vi "UNITEST MAIN v2.0.vi"() -> ()   [LabVIEW 2025]
uses:
  Traction Loop/Traction Receipe Enum.ctl
  controls/LAB-IQ UI Data.ctl
  <vilib>/Platform/TimedLoop/XDataNode/timing_clust.ctl
  <vilib>/Platform/TimedLoop/XDataNode/nitl_modes.ctl
  <vilib>/Platform/TimedLoop/XDataNode/wakeup.ctl
  HEAVE vi's/Heave Write enum.ctl
  SWAY vi's/Sway Write enum.ctl
  Traction Loop/Traction Write enum.ctl
  Acquostics Loops/Write Main Enum.ctl
  SWAY vi's/Sway Right enum.ctl
  HEAVE vi's/Heave Right enum.ctl
  Traction Loop/Traction Read enum.ctl
  Acquostics Loops/Read Main Enum.ctl
  0f9b3d6c-7caf-4790-9f98-5fac89a3677b.vi
  48f5795f-33f4-4366-aaa7-704d1097ecc1.vi
  d081153b-36ca-4bc4-8478-749476f82ba4.vi
  1202965f-721d-4349-8d61-5de826f379ef.vi
  785ec975-e53d-4ed4-be48-2cc128d7a91f.vi
  02c5850b-52e8-4ed5-91f8-6f0ad62f4994.vi
  1223eb78-e4c4-4b69-bf80-185c82055158.vi
  e5651a45-6a49-4a3f-b503-ff1eaf449b4a.vi
  <vilib>/Utility/error.llb/Trim Whitespace One-Sided.vi
  support/Message Queue/Enqueue Message (Single).vi
  <vilib>/Utility/error.llb/Error Cluster From Error Code.vi
  <vilib>/Utility/file.llb/Read Delimited Spreadsheet (string).vi
  <vilib>/Utility/file.llb/Write Delimited Spreadsheet (string).vi
  <vilib>/ErrorRing/Error Ring.xnode
  <vilib>/platform/TimedLoop/XDataNode/XDataNode.xnode
  support/Message Queue/LAB-IQ Message Queue.lvlib
  support/User Event - Stop/LAB-IQ User Event - Stop.lvlib
  <vilib>/Platform/TimedLoop/XDataNode/XDNodeRunTimeDep.lvlib
panel:
  in  "Uplink Traction":refnum<vi>
  in  "Traction":bool
  in  "Scratch":bool
  in  "LRM CAM":bool
  in  "Sway LRM":bool
  in  "Rotary Horizontal":bool
  in  "Rotary Vertical":bool
  in  "Load Cell 2":refnum<vi>
  out "AE Ring-Down Counts":u32(graph)
  out "Signal Energy":sgl(graph)
  out "Amplitude db_AE":sgl(graph)
  out "Peak Amplitude":sgl(graph)
  out "SET entrainment Velocity":dbl
  out "Test Array Size":i32
  in  "SRR INDEX [ STRIBECK]":i32
  out "Stribeck Size":i32
  out "SET SRR":dbl
  out "Enum - READ":T1
  out "ELAPSED TIMER":dbl
  out "BALL SET RPM":dbl
  out "DISC SET RPM":dbl
  out "SET LOAD":dbl
  in  "TEMPERATURE READ":dbl=40.0
  out "SET TEMPERATURE":dbl
  out "Traction Size":i32
  out "DISC SPEED (rpm)":dbl=100.0 min=0.1 max=3000.0 step=0.1 format="%.1f"
  out "BALL SPEED (rpm)":dbl=100.0 min=0.1 max=3000.0 step=0.1 format="%.1f"
  in  "BALL WEAR TRACK":dbl=7.9
  in  "DISC WEARTRACK":dbl=24.0
  in  "SRR INDEX [ TRACTION]":i32
  in  "Start Index Type":i32
  in  "Enum - Menu":T1
  out "Ball (mm/sec)":dbl
  out "Disc (mm/sec)":dbl
  in  "Traction Receipe Update Details":bool
  in  "HomeTraction":bool
  in  "Demo Mode Display":enum32{"Page 1", "Page 2"}(tab)
  in  "Traction Message":string="Recommended motion directions \nfor traction module.\n\nBall:  Counterclockwise\nDisc: Clockwise"
  in  "Traction Step Update Details":bool
  in  "Main Tab sequence for selection":T2(tab)
  out "ExceedDiscSpeed  Cinstant Speed":string
  out "ExceedBallSpeed Constant":string
  in  "TEST SELECTION (MTM) 2":enum32{"Ball Speed", "Disc Speed"}(radio)
  in  "SPEED SELECTION : MTM 2":enum32{"Speed in Rpm", "Speed in m/sec"}(radio)=enum."Speed in m/sec"
  in  "MTM Test Selection 2":enum32{"Time", "Cycle"}(radio)
  in  "Enter the Speed (m/sec):":dbl=0.5 min=3e-06 max=2500.0 step=0.001 format="%.6f"
  in  "Enter the Speed (m/sec):":dbl=0.5 min=3e-06 max=3000.0 step=0.001 format="%.6f"
  in  "Enter the Speed (RPM):":dbl=100.0 min=0.1 max=3000.0 step=0.1 format="%.1f"
  out "Lower Spped":string
  out "Upper":string
  in  "Enter the Speed (RPM):":dbl=1.0 min=0.1 max=2500.0 step=0.1 format="%.1f"
  out "ExceedBallSpeed step":string
  out "ExceedDiscSpeed":string
  out "Disc Speed Indicator":bool
  out "ExceedBallSpeed":string
  out "BallSpeed Exceed Indication":bool
  in  "Apply":bool
  in  "SPEED SELECTION : MTM":enum32{"Speed in Rpm", "Speed in m/sec"}(radio)=enum."Speed in m/sec"
  in  "TEST SELECTION (MTM)":enum32{"Ball Speed", "Disc Speed"}(radio)
  in  "MTM Test Selection":enum32{"Time", "Cycle"}(radio)
  in  "File Path Tab":enum32{"Page 1", "Page 2"}(tab)
  in  "File Path String":string="File Path Location : C:-->LAB-IQ 150 --> User Defined\n                                       Protocol-->File.txt"
  in  "Save":bool
  in  "Import":bool
  in  "File Path :":path
  in  "Step Sequence Indication Tab":enum32{"Page 1", "Page 2"}(tab)
  in  "Step Sequence Indication":string="Minimum 2 Steps required to perform the Speed Sequence"
  in  "Calculate Step":bool
  in  "StepTable":string[][](table)
  in  "Ramp Tab":enum32{"Page 1"}(tab)
  out "e.v/ssr":enum32{"E.V", "SSR"}(tab)
  in  "Enter Fixed SRR":dbl=1.0 min=-1.0 max=1.0 step=0.001 format="%.3f"
  in  "Enter the Final E.Velocity (m/s)":dbl=1.0 min=0.001 max=10.0 step=0.001 format="%.3f"
  in  "Enter initial E.Velocity (m/s)":dbl=2.0 min=0.001 max=10.0 step=0.001 format="%.3f"
  in  "Enter Fixed E.Velocity":dbl=1.0 min=0.001 max=2.0 step=0.001 format="%.3f"
  in  "Enter Final SRR":dbl=1.0 min=-1.0 max=1.0 step=0.001 format="%.2f"
  in  "Enter initial SRR":dbl=1.0 min=-1.0 max=1.0 step=0.001 format="%.2f"
  in  "Ball WTD":dbl=17.32 min=17.32 max=17.32 step=0.001 format="%.2f"
  in  "E.Velocity":bool caption="SRR"
  in  "Enter the Final Velocity (m/s)":dbl=1.0 min=0.001 max=2.0 step=0.001 format="%.3f"
  in  "Enter initial Velocity (m/s)":dbl=2.0 min=0.001 max=2.0 step=0.001 format="%.3f"
  out "Ramp Up   Disc":bool caption="Ramp Down"
  out "Initial DiscSpeed (RPM)":dbl=100.0 min=0.1 max=3000.0 step=0.1 format="%.1f"
  out "Final Speed (RPM)":dbl=1.0 min=0.1 max=3000.0 step=0.1 format="%.1f"
  out "Final Speed (RPM)":dbl=1.0 min=0.1 max=3000.0 step=0.1 format="%.1f"
  out "Initial Speed (RPM)":dbl=100.0 min=0.1 max=3000.0 step=0.1 format="%.1f"
  in  "Enter the Final Velocity (m/s)":dbl=1.0 min=0.001 max=2.0 step=0.001 format="%.3f"
  in  "Enter initial Velocity (m/s)":dbl=2.0 min=0.001 max=2.0 step=0.001 format="%.3f"
  out "Ramp Up":bool caption="Ramp Down"
  in  "Disc Motion Direction:":u16(ring) items=["Clockwise", "Counter Clockwise"]
  in  "Ball Motion Direction :":u16(ring) items=["Clockwise", "Counter Clockwise"]
  in  "Motion Mode:":u16(ring) items=["Uniform Rotation", "Speed Step", "Speed Ramp", "Speed Recipe"]
  in  "Wear Track Diameter (mm) 3":dbl=16.0 caption="Wear Track Diameter (mm):" min=1.0 max=20.0 step=0.01 format="%.2f"
  in  "Set WTD 2":bool
  in  "SRR Sweep Range (%)":string caption="Speed (mm/s)"
  out "Traction Receipe":i32(listbox)=-1
  in  "Total Execution Time":dbl
  in  "Total Steps":dbl
  in  "Duration / Step (s)":dbl=6.0
  in  "STRIBECK Fixed SRR List (%)":string="5,10,20,40,60,80,100"
  in  "Duration / Step (s)":dbl=6.0
  in  "SRR Sweep Range (%)":string
  in  "Speed (mm/s)":dbl=1000.0
  in  "Temperature Stages (°C)":string="40,100,140"
  in  "Load (N)":string="25"
  in  "Lubricant Name":string
  in  "Profile File Name":string
  out "error out":errorcluster
  in  "DEPTH TRIP   ENABLE":bool
  in  "DEPTH TRIP VALUE":dbl
  in  "LOAD TRIP  ENABLE":bool
  in  "LOAD TRIP VALUE":dbl
  in  "CYCLIC COF TRIP  ENABLE":bool
  in  "CYCLIC FF TRIP  ENABLE":bool
  in  "FF TRIP  ENABLE":bool
  in  "COF TRIP  ENABLE":bool
  in  "CYCLIC CoF TRIP VALUE":dbl
  in  "CYCLIC FF TRIP VALUE":dbl
  in  "FF TRIP VALUE":dbl
  in  "COF TRIP VALUE":dbl
  in  "Gain 2":dbl=0.016
  in  "Offset  3":dbl=1.5
  in  "Ramp MulFac":dbl=2.0
  out "actpid":dbl
  in  "pulses LoadDiffRamp(2..10)":dbl=9.0
  in  "PulseControlRamp(diff<=3N)":dbl=5.0 min=1.0 max=1000.0 step=1.0 format="%#.1f"
  in  "SetLoadDeadband(%) Load(0-10N)":dbl=0.1 min=0.0001 max=100.0 step=0.0001 format="%#.6f"
  in  "pulses LoadDiff(2..10)":dbl=10.0
  in  "pulses LoadDiff(11..50)":dbl=40.0
  in  "PulseControl(diff<=3N)":dbl=1.0 min=1.0 max=1000.0 step=1.0 format="%#.1f"
  out "SetLoadDeadband(%)  2":dbl=1.0 min=0.001 max=100.0 step=0.001 format="%#.6f"
  in  "pulsesSent":dbl=200.0
  out "pulses":dbl
  in  "pulses LoadDiff(21..1000)":dbl=40.0
  in  "Delay":dbl=1.5 min=0.001 max=5.0 step=0.001 format="%#.6f"
  in  "deadband":dbl=0.2
  in  "Checkbox 2":bool
  in  "Checkbox":bool=TRUE
  out "Scratch Start Recording":bool
  in  "SwaySpeed Set":bool
  in  "Update":bool
  in  "Analysis Home":bool
  in  "Installation/Replacement completed":bool
  in  "Loahead":bool
  in  "Heave and Surge COM Port:":refnum<visa-resource-name>="COM9"
  in  "Sway COM Port:":refnum<visa-resource-name>="COM10"
  out "Test Trip":bool
  out "Hymidity":bool
  in  "Humidity Disable trip":bool=TRUE
  in  "CoF Trip  2":dbl=540.0 min=100.0 max=540.0 step=1.0
  in  "File Path :  2":path
  out "Wear Track Diameter":dbl
  in  "Stribeck table":bool
  in  "seq":bool=TRUE
  out "Drive Error":string
  out "mm/s  Surge":dbl=7.0 caption="Jog" min=0.001 max=50.0 step=0.0001 format="%.2f"
  in  "Update Surge Speed":bool
  out "mm/s  Sway":dbl=7.0 caption="Jog" min=0.001 max=50.0 step=0.0001 format="%.2f"
  in  "Update Sway Speed":bool
  in  "Update Heave Speed":bool
  out "mm/s Heave":dbl=7.0 caption="Jog" min=0.001 max=30.0 step=0.0001 format="%.2f"
  in  "mm/sec":dbl=1.0 caption="Jog" min=0.001 max=50.0 step=0.001 format="%.2f"
  out "Scratch Start Test":bool
  in  "HomeScratch":bool
  in  "TEST SELECTION":enum32{"Time", "Cycle"}(radio)
  out "Spare 15":u8
  out "Spare 14":u8
  out "Spare 13":u8
  out "Spare 12":u8
  out "Spare 11":u8
  out "Spare 10":u8
  out "Spare 9":u8
  out "Spare 8":u8
  out "Start Test Temp":bool
  in  "AppLoadSeq scratch":bool
  in  "PID Delay (sec)":dbl=1.0 format="%#_6p"
  out "Spare 15":u8
  out "Spare 14":u8
  out "Spare 13":u8
  out "Spare 12":u8
  out "Spare 11":u8
  out "Spare 10":u8
  out "Spare 9":u8
  out "Spare 8":u8
  out "Load Cell Temp":bool
  in  "Stop Scratch":bool
  in  "Enter Fixed SRR 2":dbl min=0.0 max=0.0 format="%.3f"
  in  "E.Velocity 2":bool=TRUE caption="SRR"
  in  "Tab Control 3":T3(tab)
  in  "Tab Control 14":T4(tab)=enum."Motor Load"
  in  "Ramp":bool
  in  "PID":T5={"min_deadband_floor"=50000000.0, "min_finetune_floor"=10.0, "dynamic_spindle_noise_scalar"=100.0, "filter_alpha"=0.05, "Vertical load (N)"=0.0, "Pulse delta"=0.0, "Fine Tune Zone"=10.0, "Max_pos_limit"=50000000.0, "Min_pos_limit"=0.0, "i_limit"=10.0, "Max Step Linit"=10.0, "Init Step"=10.0, "pct_scale"=100.0, "Deadband"=0.1, "Kd"=0.0, "Ki"=0.0, "Kp"=1.0, "Current Position"=0.0, "Set Load"=0.0, "Current Load"=0.0, "gFF Rot 7"={0.0, 0.0, 0.0}, "Bypass Load"=FALSE, "Enter ByPass Load"=0.0, "apply load"=FALSE} {"Vertical load (N)" format="%#.3f"}
  in  "deleteHandle-result":i32
  in  "initial-return":i32
  in  "filter-return":i32
  in  "zero-return":i32
  in  "get-range-return":i32
  in  "get-data-return":i32
  in  "ft_udp_handle":i32
  in  "AE":bool
  in  "reinit 3":bool=TRUE
  in  "AutoTune":bool
  in  "Dummy Run":bool
  in  "running_flag":bool
  in  "Create Handle":bool=TRUE
  in  "delete Handle":bool
  in  "ft_range":dbl[](array[numeric])=[1.0, 1.0, 1.0, 1.0, 1.0, 1.0]
  in  "ft_data":dbl[](array[numeric])=[1.0, 1.0, 1.0, 1.0, 1.0, 1.0]
  in  "PID gains out delay (microForce)":T6={"proportional gain (Kc)"=300.0, "integral time (Ti, min)"=0.00011, "derivative time (Td, min)"=0.0} {"derivative time (Td, min)" format="%.3f"; "integral time (Ti, min)" min=1e-05 max=100.0 step=1e-06 format="%.6f"; "proportional gain (Kc)" format="%.3f"}
  in  "PID gains out delay":T6={"proportional gain (Kc)"=30.0, "integral time (Ti, min)"=0.00101, "derivative time (Td, min)"=0.0} {"derivative time (Td, min)" format="%.3f"; "integral time (Ti, min)" min=1e-05 max=100.0 step=0.0001 format="%.4f"; "proportional gain (Kc)" format="%.3f"}
  in  "output range delay":cluster{"output high":dbl, "output low":dbl}={"output high"=100.0, "output low"=-100.0} {"output low" format="%.2f"; "output high" format="%.2f"}
  in  "Load(N)":dbl[](array[numeric])
  in  "FFy(N)":dbl[](array[numeric])
  in  "FFx(N)":dbl[](array[numeric])
  in  "Mx(Nm)":dbl[](array[numeric])
  in  "My(Nm)":dbl[](array[numeric])
  in  "Mz(Nm)":dbl[](array[numeric])
  in  "Port":i32=8080
  in  "Sensor IP":string="192.168.1.100"
  in  "SN":i32
  in  "model":string
  in  "Burst Delay (ms)":dbl=10.0
  in  "Acq Delay (ms)":dbl=10.0
  in  "ZeroAll":bool
  in  "ClearAll":bool
  in  "Save Dwell":dbl=0.015 caption="Save Dwell (sec)" min=0.0 max=5.0 step=0.001 format="%.3f"
  out "TORQUE (N-m)":dbl[][](graph)
  out "FORCE (N)":dbl[][](graph)
  in  "stop 6":bool
  in  "Tab Control 19":enum32{"Platform COM", "Config ", "DevInfo"}(tab)=enum."Config "
  in  "Manual Write Acquostic":bool
  out "data out":string
  out "Last Config Rejected":u32
  out "rx command count":u32
  out "Current Filter Id":u32
  out "Isolated Gain":u32
  out "DAQ Status":u32
  out "Heave and Surge Read":string
  out "error out Write":errorcluster
  out "error out Read":errorcluster
  out "Read Heave Temp":bool
  out "Heave and Surge Write":string
  in  "Manual Write Heave & Surge":bool
  out "HEAVE ENABLE":bool
  out "SWAY READ":string
  out "error out Write  SWAY":errorcluster
  out "error out Read SWAY":errorcluster
  out "Read SWAY Temp":bool
  out "SWAY WRITE":string
  in  "Manual Write SWAY":bool
  out "TRACTION READ":string
  out "error out Write  TRACTION":errorcluster
  out "error out Read TRACTION":errorcluster
  out "Read TRACTION Temp":bool
  out "TRACTION WRITE":string
  in  "Manual Write TRACTION":bool
  in  "Uplink Packet":T7
  out "Downlink Packet":T8
  in  "error in (no error)":errorcluster
  out "error out":errorcluster
  in  "UPLINK HEAVE":T9={"Sequence ID"=0, "Mode Command"=2, "Distance"=10000.0, "SPEED"=10000.0, "Reserved"=0.0, "SPARE 1"=0, "SPARE 2"=0, "SPARE 3"=0, "SPARE 4"=0, "SPARE 5"=0, "SPARE 6"=0, "SPARE 7"=0, "SPARE 8"=0, "SPARE 9"=0, "SPARE 10"=0, "SPARE 11"=0, "SPARE 12"=0, "SPARE 13"=0, "SPARE 14"=0, "SPARE 15"=0, "SPARE 16"=0, "SPARE 17"=0}
  out "DOWNLINK HEAVE":T10 {"HEAVE POSE" format="%#.6f"; "SURGE POSE" format="%#.6f"; "Missed Packets" format="%#.6f"}
  in  "UPLINK SWAY":T11={"Sequence ID"=0, "Mode Command"=2, "Distance"=10000.0, "SPEED"=10000.0, "Reserved"=0.0, "SPARE1"=0, "SPARE 2"=0, "SPARE  3"=0, "SPARE  4"=0, "SPARE  5"=0, "SPARE 6"=0, "SPARE 7"=0, "SPARE 8"=0, "SPARE 9"=0, "SPARE 10"=0, "SPARE 11"=0, "SPARE 12"=0, "SPARE 13"=0, "SPARE 14"=0, "SPARE 15"=0, "SPARE 16"=0, "SPARE 17"=0}
  out "DOWNLINK SWAY":T12 {"SWAY POSE" format="%#.6f"; "Rotary POSE" format="%#.6f"; "Missed Packets" format="%#.6f"}
  in  "Uplink Traction":T13={"Sequence ID"=0, "Mode Command"=2, "Distance"=10000.0, "SPEED"=10000.0, "Reserved "=0.0, "SPARE 1"=0, "SPARE 2"=0, "SPARE  3"=0, "SPARE  4"=0, "SPARE  5"=0, "SPARE 6"=0, "SPARE 7"=0, "SPARE 8"=0, "SPARE 9"=0, "SPARE 10"=0, "SPARE 11"=0, "SPARE 12"=0, "SPARE 13"=0, "SPARE 14"=0, "SPARE 15"=0, "SPARE 16"=0, "SPARE 17"=0}
  out "Downlink traction":T14 {"TRACTION POSE 1" format="%#.6f"; "TRACTION POSE 2" format="%#.6f"; "Missed Packets" format="%#.6f"}
  in  "JOG TRIP LOAD VALUE (N)":dbl
  in  "SAMPLES":dbl=100.0
  in  "Re-initilaize":bool
  in  "Filter ON/OFF":bool=TRUE
  in  "TracHomeSurgeOffsetCounts 10MM":dbl=505100.0
  in  "TracHomeSwayOffsetCounts 10MM":dbl=1432.0
  in  "Acoustic Emission:":dbl=1.0 min=0.0001 max=200.0 step=0.0001 format="%.4f"
  in  "Apply Filter (FF)":bool
  in  "Filter% 2":dbl=50.0 min=50.0 max=100.0 step=0.1 format="%.1f"
  in  "Apply Filter (Load)":bool=TRUE
  in  "Filter%":dbl=80.0 min=50.0 max=100.0 step=0.1 format="%.1f"
  in  "Sway distance (mm)":dbl=245.0
  in  "Surge distance (mm)":dbl=370.0
  in  "DataSavingLoopDelay(ms)":dbl=15.0
  in  "SAVE  2":bool
  in  "Enter Distance":bool caption="Enter Counts"
  in  "Sway Counts:":dbl=100.0 min=0.0 max=100000000.0 step=1.0 format="%.2f"
  in  "Distance (mm): 3":dbl=100.0 caption="Distance (mm):" min=0.0 max=1500.0 step=0.001 format="%.5f"
  in  "Surge Counts:":dbl=100.0 min=0.0 max=100000000.0 step=1.0 format="%.1f"
  in  "Distance (mm): 2":dbl=100.0 caption="Distance (mm):" min=0.0 max=1500.0 step=0.0001 format="%.3f"
  in  "Distance (mm):":dbl=100.0 min=0.0 max=1500.0 step=0.001 format="%.5f"
  in  "Heave Counts:":dbl=100.0 min=0.0 max=100000000.0 step=1.0
  in  "LRMHomeSurgeOffsetCounts":dbl=307197.0
  in  "LRMHomeSwayOffsetCounts":dbl=26880.0
  in  "TracHomeSurgeOffsetCounts 20MM":dbl=505100.0
  in  "TracHomeSwayOffsetCounts 20MM":dbl=1432.0
  in  "RotHomeSwayOffsetCounts":dbl=14656.0
  in  "RotHomeSurgeOffsetCounts":dbl=311465.0
  in  "Heave distance":dbl=340.0
  out "Zmm":dbl=1600.0
  out "Heave Pulses/mm":dbl=1600.0
  out "Surge Pulses/mm":dbl=1600.0
  out "Sway Pulses/mm":dbl=320.0
  in  "Heave Pitch":dbl=4.0
  in  "Surge Pitch":dbl=3.0
  in  "Sway Pitch":dbl=2.0
  in  "Heave PPR":dbl=6400.0
  in  "Surge PPR":dbl=6400.0
  in  "Sway PPR":dbl=6400.0
  in  "Heave Jog Speed":dbl=15.0
  in  "Surge Jog Speed":dbl=1.0 format="%.4f"
  in  "Heave PID Speed":dbl=15.0
  in  "Heave Loop Delay":dbl
  in  "Sway Jog Speed":dbl=1.0 format="%.4f"
  in  "Sway PID Speed":dbl=1.0 format="%.4f"
  in  "Sway Loop Delay":dbl
  in  "GUI":T15(tab)
  in  "Platform Settings":bool caption="Password"
  in  "Configure":bool caption="Password"
  in  "Home":bool caption="Password"
  in  "EXIT":bool
  in  "Analysis":bool caption="Password"
  in  "service 2":bool caption="Password"
  in  "MainPage":T16(tab)=enum."HOME"
  in  "Select Load Head":bool
  in  "Notes :":string
  in  "FILE":string
  in  "Sample ID :":string
  in  "Operator ID :":string
  in  "Operator Name :":string
  in  "Auto":bool caption="Power Status"
  in  "Disable Axis Jog Soft Limits m":bool
  out "Sway and Surge COM Status":bool=TRUE caption="Load COM Status"
  out "Heave COM Status":bool=TRUE caption="Load COM Status"
  in  "Enable Platform":bool
  in  "Surge Forward Main":bool
  in  "Surge Backward Main":bool
  in  "Sway Right Main":bool
  in  "Sway Left Main":bool
  in  "Heave Down Main":bool
  in  "Heave Up main":bool
  in  "mm":dbl=0.001 caption="Jog" min=0.001 max=30.0 step=0.01 format="%#.3f"
  in  "Surface Analysis":bool
  in  "Imaging":bool
  in  "Image Analysis":bool
  in  "Post Analysis":bool
  in  "SSP 0.75":bool
  in  "SSP 0.5":bool
  in  "SSP 0.3":bool
  in  "Warning":enum32{"Page 2"}(tab)
  in  "gui GIF":enum32{"Check", "Deca", "kilo", "Micro"}(tab)
  out "Communication is established":bool=TRUE caption="Load COM Status"
  in  "Reference Sample":u16(ring) items=["None", "Brass", "Aluminium", "Mild Steel"]
  out "Load Cell Communication Slide":u8(slide)=1 min=1 max=10 step=1 scale=0.0..10.0
  in  "com 3":bool
  out "com":bool
  out "DecaForce COM Status":bool caption="Load COM Status"
  in  "Loading Mode":u16(ring) items=["Constant", "Ramp", "Steps", "Indentation"]
  in  "Enter the CoF Trip":dbl=1.0
  in  "Enter the Friction Force Trip":dbl=520.0 min=500.0 max=500.0 step=1.0 format="%#.1f"
  in  "Enter the Normal load Trip":dbl=520.0 min=500.0 max=500.0 step=0.001 format="%.3f"
  in  "KiloForce":bool
  in  "DecaForce":bool
  in  "MicroForce":bool
  in  "LHBack":bool
  in  "LHNext":bool
  in  "Load Selection":T17(tab)
  in  "Enter the Load  (N)":dbl=2.0 caption="Enter the Load (N)" min=2.0 max=50.0 step=0.1 format="%#.4f"
  in  "Enter the Final Load (N)":dbl=1.0 min=0.0 max=500.0 step=1.0 format="%#.0f"
  in  "Enter the Loading Rate (N/min)":dbl=60.0 min=1.0 max=1200.0 step=0.1 format="%.2f"
  out "Warning 2":bool
  in  "Stribeck Table  For loading":string[][](table)
  in  "Clear 3":bool
  out "Message":string="Load Entered is out of range!!!"
  in  "Indentation":string[][](table)=[["Detection", "5", "2"], ["Unload", "0", "5"], ["Load", "10", "2"], ["Unload", "0", "5"], ["Detection", "5", "2"], ["Unload", "0", "5"]]
  in  "Multipoint":bool caption="Singlepoint"
  in  "AppLoad 4":bool
  in  "zNL":bool
  out "NL disp":dbl caption="Normal Load ( N )" min=-2000.0 max=2000.0 step=0.0001 format="%.1f"
  in  "Traction":bool
  in  "Surge Forward MM":bool
  in  "Surge Backward MM":bool
  in  "M3 Image":enum32{"Page 1", "Page 2"}(tab)
  in  "String 39":string="Jog heave to bring the upper sample closer to the lower sample within 1mm."
  in  "Sway Left MM":bool
  in  "Sway Right MM":bool
  in  "Disable Axis Jog Soft Limits":bool
  in  "mm":dbl=0.001 caption="Jog" min=0.001 max=5.0 step=0.0001 format="%#.3f"
  in  "Heave Down MM":bool
  in  "Heave Up MM":bool
  in  "Wear Track Diameter (mm)":dbl=30.0 caption="Wear Track Diameter (mm):" min=1.0 max=30.0 step=1.0 format="%.2f"
  in  "Set WTD":bool
  in  "HomeScratch":bool
  in  "HomeRot":bool
  in  "PlaceModule":bool
  in  "Motion Mode:":u16(ring) items=["Uniform Rotation", "Angular Oscillation", "Stribeck ", "Steps"]
  in  "LR Sway":bool
  in  "Rot Hor":bool
  in  "Rot Ver":bool
  in  "Scratch":bool
  in  "LR Cam":bool
  in  "MMBack":bool
  in  "MMNext":bool
  in  "Rotary Module Selection":T18(tab)
  in  "SPEED SELECTION :":enum32{"Speed in RPM", "Speed in m/sec"}(radio)=enum."Speed in m/sec"
  in  "Enter the Speed(mm/sec)":dbl=0.1 min=0.0001 max=1000.0 step=0.1 format="%#.4f"
  in  "Enter the Speed (RPM)":dbl=45.0 min=1.0 max=3000.0 step=1.0
  in  "Enter the Frequency (Hz)":dbl=1.0 min=0.1 max=10.0 step=0.1 format="%.1f"
  in  "Enter the Angle (Deg)":dbl=45.0 min=5.0 max=300.0 step=1.0
  in  "Angular Oscillation Set":bool
  in  "Rotary Tab":enum32{"Page 1", "Page 2"}(tab)
  out "e.v/ssr 2":enum32{"E.V", "SSR"}(tab)
  in  "Enter the Final E.Velocity (m/s) 2":dbl=1.0 min=0.001 max=4.0 step=0.001 format="%.3f"
  in  "Enter initial E.Velocity (m/s) 2":dbl=2.0 min=0.001 max=4.0 step=0.001 format="%.3f"
  in  "Enter Fixed E.Velocity 2":dbl=1.0 min=0.001 max=2.0 step=0.001 format="%.3f"
  in  "Enter Final SRR 2":dbl=1.0 min=0.001 max=1.0 step=0.001 format="%.2f"
  in  "Enter initial SRR 2":dbl=1.0 min=0.001 max=1.0 step=0.001 format="%.2f"
  out "Final Speed (RPM) 3":dbl=1.0 min=0.1 max=3000.0 step=0.1 format="%.1f"
  out "Initial Speed (RPM) 2":dbl=100.0 min=0.1 max=3000.0 step=0.1 format="%.1f"
  in  "Enter the Final Velocity (m/s) 3":dbl=1.0 min=0.001 max=2.0 step=0.001 format="%.3f"
  in  "Enter initial Velocity (m/s)  3":dbl=2.0 min=0.001 max=2.0 step=0.001 format="%.3f"
  out "Ramp Up 2":bool caption="Ramp Down"
  in  "Import 2":bool
  in  "Save 2":bool
  in  "SPEED SELECTION : rotary":enum32{"Speed in Rpm", "Speed in m/sec"}(radio)=enum."Speed in m/sec"
  in  "calculate rotary":bool
  in  "String 45":string="File Path Location : C:-->LAB-IQ 150 --> User Defined\n                                       Protocol-->File.txt"
  in  "Step Speed":enum32{"Step Speed", "Step (load-Speed)"}(tab)
  in  "StepTable For Speed":string[][](table)
  in  "StepTable For Load-Speed":string[][](table)=[["", "", ""], ["", "", ""], ["", "", ""], ["", "", ""]]
  in  "StepTable For Speed 3":string[][](table)=[["", "", ""], ["", "", ""], ["", "", ""], ["", "", ""]]
  in  "Motion Direction:  3":u16(ring) items=["Clockwise", "Counter Clockwise"]
  in  "Enter Scratch length (mm):":dbl=1.0 min=1.0 max=50.0 step=0.0001 format="%.4f"
  in  "Enter Scratch Speed (mm/s):":dbl=1.0 min=0.003 max=10.0 step=0.0031 format="%.5f"
  in  "Scartch Offset":dbl=1.0 caption="Scratch Offset: (mm)" min=0.1 max=5.0 step=0.1 format="%.1f"
  in  "Motion type:":u16(ring) items=["Unidirection", "Bidirection"]
  in  "Scratch Mode":u16(ring) items=["Scratch", "Pre-Post Scan", "Multi Scratch"]
  in  "Rotary Speed Exced":string="Motor Speed Out of Range"
  in  "No of Scratch":dbl=1.0 min=1.0 max=50.0 step=0.0001
  out "Humidity  Status  3":bool caption="Communication Status"
  out "Low Temp  Status  2":bool=TRUE caption="Communication Status"
  out "TK4 status 2":bool=TRUE caption="Communication Status"
  in  "Acuostic M":string="Before selecting Acoustic make sure the sensor output pin is connected to A4."
  in  "Stage Temperature":dbl[](array[numeric])=[150.0, 230.0, 300.0, 350.0, 400.0, 450.0, 500.0]
  in  "Sample Temperature":dbl[](array[numeric])=[100.0, 150.0, 200.0, 250.0, 300.0, 350.0, 400.0]
  in  "Humidity (Amb)":bool
  in  "Clear List":bool
  out "Sensors Picked":string
  in  "Add to list":bool
  in  "Wear":bool
  in  "Vibration":bool
  in  "Humidity (Chamber)":bool
  in  "Temperature (Chamber)":bool
  in  "ECR":bool
  in  "Temperature (Amb)":bool
  in  "Microphone":bool
  in  "Acoustic Emission 3":bool
  in  "SNext":bool
  in  "APBack":bool
  in  "Enter the Temperature (°C):":dbl
  in  "Enter the Stage \nTemperature (°C):":dbl=20.0 min=20.0 max=150.0 step=1.0 format="%#.0f"
  in  "Enter the Humidity (%Rh):":dbl=30.0 min=30.0 max=85.0 step=1.0
  in  "Low Temp":bool
  in  "High Temp":bool
  in  "Humidity":bool
  in  "Gains":enum32{"20dB", "40dB", "60dB"}(radio)=enum."60dB"
  in  "Main Screen Tab":T19(tab)
  in  "Depth Reset Graph":bool
  out "Weart Deapth":bool
  in  "Depth Trip 2":bool=TRUE
  out "Depth Trip":dbl=600.0
  out "NL Display 4":dbl caption="Normal Load ( N )" min=-2000.0 max=2000.0 step=0.0001 format="%.1f"
  in  "Load Reset Graph":bool
  in  "Load Disable Trip":bool=TRUE
  out "Load pid":bool
  out "NL Trip 2":dbl=600.0
  in  "ClrLog":bool
  out "Trip Log":string
  in  "Start Test":bool
  out "Test status":bool caption="Test Status"
  out "AR Led":bool caption="AR"
  out "Data":bool=TRUE
  out "Health":bool=TRUE
  out "Sway COM Status":bool=TRUE caption="Load COM Status"
  out "Heave COM Status":bool=TRUE caption="Load COM Status"
  in  "BACK":bool
  out "Ambient \nTemperature":dbl min=0.0 max=5000.0 step=0.1 format="%.1f"
  out "Ambient\n Humidity":dbl min=0.0 max=5000.0 step=0.1 format="%.2f"
  out "NL disp 2":dbl caption="Normal Load ( N )" min=-2000.0 max=2000.0 step=0.0001 format="%.1f"
  out "Set Humidity":dbl caption="Set Humidity  (% Rh)" min=-2000.0 max=2000.0 step=1.0 format="%.1f"
  out "humidity disp":dbl caption="Humidity (% Rh)" min=-2000.0 max=2000.0 step=1.0 format="%.1f"
  in  "Humidity On":bool
  in  "zNL 2":bool
  out "NLt":bool
  in  "Load En":bool
  out "Freq (Hz)":dbl min=0.0 max=5000.0 step=0.1 format="%.4f"
  out "HumCOMStatus":bool caption="Communication Status"
  out "Load Communication":bool
  in  "Temp Tabs":enum32{"Low Temp", "High Temp"}(tab)=enum."High Temp"
  out "Controller  Status":bool
  out "ChamberTemp":dbl format="%#.1f"
  in  "SetTmp":dbl=-190.0 caption="Set Temperature (Deg C)" min=-190.0 max=100.0 step=1.0 format="%.1f"
  in  "Cooling":bool
  in  "Heater":bool
  out "TK4 status":bool caption="Controller  Status"
  out "ChamberTemp":dbl format="%#.1f"
  in  "SetTmp":dbl caption="Set Temperature (Deg C)" min=0.0 max=1000.0 step=1.0 format="%.1f"
  in  "Set Load (N)":dbl=100.0 min=0.01 max=1500.0 step=0.01 format="%.1f"
  in  "Time Tab":enum32{"cycles", "duration"}(tab)=enum."duration"
  out "Test Duration 4":dbl=600.0 caption="Test Duration\n(HH:MM:SS)" min=0.0083 max=180000.0 step=0.0001 format="%<%H:%M:%S>t"
  out "TEST CYCLE":dbl min=0.0 max=5000.0 step=0.01 format="%.2f"
  in  "TOTAL CYCLES":dbl min=0.0 max=5000.0 step=0.1 format="%.4f"
  out "Time ( HH:MM:SS ) 2":dbl min=0.0 max=144000.0 step=1.0 format="%<%H:%M:%S>t"
  in  "Test Duration":dbl=600.0 caption="Test Duration\n(HH:MM:SS)" min=0.0083 max=180000.0 step=0.0001 format="%<%H:%M:%S>t"
  in  "Main Speed Tab":enum32{"ROTARY", "TRACTION"}(tab)
  in  "SPEED TAB":enum32{"RPM", "m/sec"}(tab)
  out "Speed (RPM)":dbl min=0.0 max=5000.0 step=0.1 format="%.1f"
  out "Set Speed":dbl caption="Set Speed (RPM)" min=0.0 max=1500.0 step=0.1 format="%.1f"
  out "Speed (m/sec)":dbl min=0.0 max=5000.0 step=0.001 format="%.4f"
  out "Set Speed (m/sec)":dbl min=0.0 max=1500.0 step=0.001 format="%.4f"
  in  "MTM MOTOR DISPLAY":enum32{"MTM RPM", "MTM m/sec"}(tab)
  out "Disc Speed (RPM)":dbl min=0.0 max=1500.0 step=0.1 format="%.1f"
  out "Ball Speed (RPM)":dbl min=0.0 max=1500.0 step=0.1 format="%.1f"
  out "Disc Speed (m/sec)":dbl min=0.0 max=1500.0 step=0.1 format="%.1f"
  out "Ball Speed (m/sec)":dbl min=0.0 max=1500.0 step=0.1 format="%.1f"
  in  "Angle and Frequency":enum32{"angular", "lrm"}(tab)
  out "Angle (Deg)":dbl min=0.0 max=5000.0 step=0.01 format="%.2f"
  out "Stroke (mm)":dbl min=0.0 max=5000.0 step=0.01 format="%.2f"
  in  "STOP":bool
  out "Multi Scratch Pass":dbl min=0.0 max=5000.0 step=0.1
  in  "FF Tab":T20(tab)
  in  "COF Reset Graph":bool
  in  "COF Disable Trip":bool=TRUE
  out "COF TRIP":dbl=600.0
  out "Coefficient of Friction":dbl(graph)=0.13298760003255525
  in  "zFF":bool
  out "Friction Force (N)":dbl min=-2000.0 max=2000.0 step=0.0001 format="%.3f"
  in  "FF Reset Graph":bool
  in  "FF Disable Trip":bool=TRUE
  out "FF TRIP":dbl=600.0
  out "Friction Force (N) Graph":dbl(graph)=0.13298760003255525
  in  "CZ FF":bool
  out "Cyclic Friction Force (N)":dbl min=-2000.0 max=2000.0 step=0.0001 format="%.3f"
  out "Cyclic FF TRIP":dbl=600.0
  in  "Cyclic FF Disable Trip":bool=TRUE
  in  "Cyclic FF Reset Graph":bool
  out "Cyclic Friction Force (N) Graph":dbl(graph)=0.13298760003255525
  out "cyclic COF TRIP":dbl=600.0
  in  "cyclic COF Disable Trip":bool=TRUE
  in  "cyclic COF Reset Graph":bool
  out "Cyclic Coefficient of Friction":dbl(graph)=0.13298760003255525
  out "Main Chart 3":cluster{dbl, "NL disp":dbl, dbl}(graph)
  out "WearGp":dbl(graph)=0.13298760003255525
  out "Depth (µm)":dbl min=-200.0 max=200.0 step=0.1 format="%.1f"
  in  "Depthz":bool
  out "Weart":bool
  in  "Sub Graph":T21(tab)
  in  "Speed Tab":enum32{" Rotary Disc", "MTM Ball", "MTM Disc"}(tab)
  in  "Speed Reset Graph":bool
  out "speed mm/sec":dbl(graph)=0.13298760003255525
  out "MTM BALL SPEED":dbl(graph)=0.13298760003255525
  out "MTM DISC  SPEED":dbl(graph)=0.13298760003255525
  in  "Temperature Reset":bool
  out "Temperature (deg c)":dbl(graph)=0.13298760003255525
  out "ECR 2":dbl(graph)=0.13298760003255525
  in  "ECR RESET":bool
  out "Acoustic Emission (mV)":dbl min=0.0 max=5000.0 step=0.1
  in  "Aqucostic Reset Graph":bool
  out "gACQUOS":dbl(graph)=0.13298760003255525
  in  "Humidity Reset Graph":bool
  out "HumrGp":dbl(graph)=0.13298760003255525
  out "SD (mm)":dbl caption="Sliding Distance ( mm )" min=-200.0 max=200.0 step=0.1 format="%.4f"
  in  "Siliding distance Reset Graph":bool
  out "SDGp":dbl(graph)=0.13298760003255525
  in  "X-AXIS":u16(ring) items=["None", "Time ( Sec )", "Normal Load ( N )", "Frictional Force ( N )", "Coefficient of Friction", "Depth ( Microns )", "Speed ( RPM )", "Frequency ( Hz )", "Angle ( Degree )", "Cyclic Friction Force ( N )", "Cyclic Co efficient Friction ", "Stage temperature ( Degree celcius )", "Sample temperature ( Degree celcius )", "Stroke Length ( mm )", "Scratch Speed ( mm/sec )", "Amb Humidity ( % Rh ) ", "Amb Temperature (Deg C)", "Acoustic (mV)", "Mx (Nm)", "My (Nm)", "Mz (Nm)", "Humidity ( % Rh )", "Sliding Distance (mm)", "Wear Track Diameter (mm)", "Fx(N)", "Fy(N)", "MTM BallSpeed (RPM)", "MTM DiscSpeed (RPM)", "Entrainment Speed", "Slide Role", "Slip(%)", "Rotary Speed (m/sec)", "MTM Ball Speed (m/sec)", "MTM Disc Speed (m/sec)", "ECR (ohms)"]
  in  "Y-AXIS":u16(ring) items=["None", "Time ( Sec )", "Normal Load ( N )", "Frictional Force ( N )", "Coefficient of Friction", "Depth ( Microns )", "Speed ( RPM )", "Frequency ( Hz )", "Angle ( Degree )", "Cyclic Friction Force ( N )", "Cyclic Co efficient Friction ", "Stage temperature ( Degree celcius )", "Sample temperature ( Degree celcius )", "Stroke Length ( mm )", "Scratch Speed ( mm/sec )", "Amb Humidity ( % Rh ) ", "Amb Temperature (Deg C)", "Acoustic (mV)", "Mx (Nm)", "My (Nm)", "Mz (Nm)", "Humidity ( % Rh )", "Sliding Distance (mm)", "Wear Track Diameter (mm)", "Fx(N)", "Fy(N)", "MTM BallSpeed (RPM)", "MTM DiscSpeed (RPM)", "Entrainment Speed", "Slide Role", "Slip(%)", "Rotary Speed (m/sec)", "MTM Ball Speed (m/sec)", "MTM Disc Speed (m/sec)", "ECR (ohms)"]
  out "XY Graph":cluster{"Array 2":dbl[], "Array 2":dbl[]}[](graph) caption="XY Graph 20"
  out "VARIANCE":dbl=-0.0 format="%0.2f"
  out "SD":dbl=-0.0 format="%.3f"
  out "MEAN":dbl format="%.3f"
  out "VARIANCE":dbl=-0.0 format="%0.2f"
  out "SD":dbl=-0.0 format="%.3f"
  out "MEAN":dbl format="%.3f"
  out "VARIANCE":dbl=-0.0 format="%0.2f"
  out "SD":dbl=-0.0 format="%.3f"
  out "MEAN":dbl format="%.3f"
  out "VARIANCE":dbl=-0.0 format="%0.2f"
  out "SD":dbl=-0.0 format="%.3f"
  out "MEAN":dbl format="%.3f"
  in  "Analysis Home new":bool
  out "File 2 Discription":string="\r"
  out "File 1 Discription":string="\r"
  in  "OPEN 1":bool
  in  "OPEN 2":bool
  out "File Name 1":string
  out "File Name 2":string
  in  "Refresh 2":bool
  in  "OPEN 3":bool
  out "File Name 3":string
  out "File Name 4":string
  in  "OPEN 4":bool
  out "File 4 Discription":string="\r"
  out "File 3 Discription":string="\r"
  in  "File Format":u16(ring) items=["csv", "txt", "duf"]
  in  "Export":bool
  in  "Report":bool
  in  "Password":string
  in  "Home Service":bool
  in  "Advanced Setting":bool
  in  "About Tab":enum32{"Primary"}(tab)
  in  "ECR Port:":refnum<visa-resource-name>="COM10"
  in  "Ramp Port:":refnum<visa-resource-name>="COM10"
  in  "Temp Modbus:":refnum<visa-resource-name>="COM14"
  in  "Humidity Port:":refnum<visa-resource-name>="COM10"
  in  "Edit Gain Constants":bool
  in  "Save Gain Constants":bool
  in  "Service About":bool
  # "1. Test Identification & Global Setup"
  # "2. Step Configurations & Timing"
  # "Step 1 Configuration: TRACTION Step"
  # "SET JOG SPEED"
  # "%"
  # "NOTE: This operation needs to be done only when the machine is ON."
  # "Steps 2+ Configuration: STRIBECK Steps"
  # "Upper Drive (Ball)"
  # "Lower Drive (Disc)"
  # "Variable"
  # "Configuration"
  # "Limits for Heave Surge and Sway"
  # "Modules Offset Parameters"
  # "Counts-Distance Calculator"
  # "File Name :"
  # "Ensure the traction module is aligned\n horizontally with the stage before ENABLE."
  # "JOG MODE"
  # "Module Selection"
  # "Positioning Control"
  # "Connect the controller\ncable to M3"
  # "Environment"
  # "Sensors"
  # "Data Points"
  # "Data Points"
  # "Data Points"
  # "Data Points"
  # "Data Points"
  # "Data Points"
  # "Data Points"
  # "LAB-IQ 150 / UNITEST / WO2479 / UT150  v05 / AUGUST 2026"
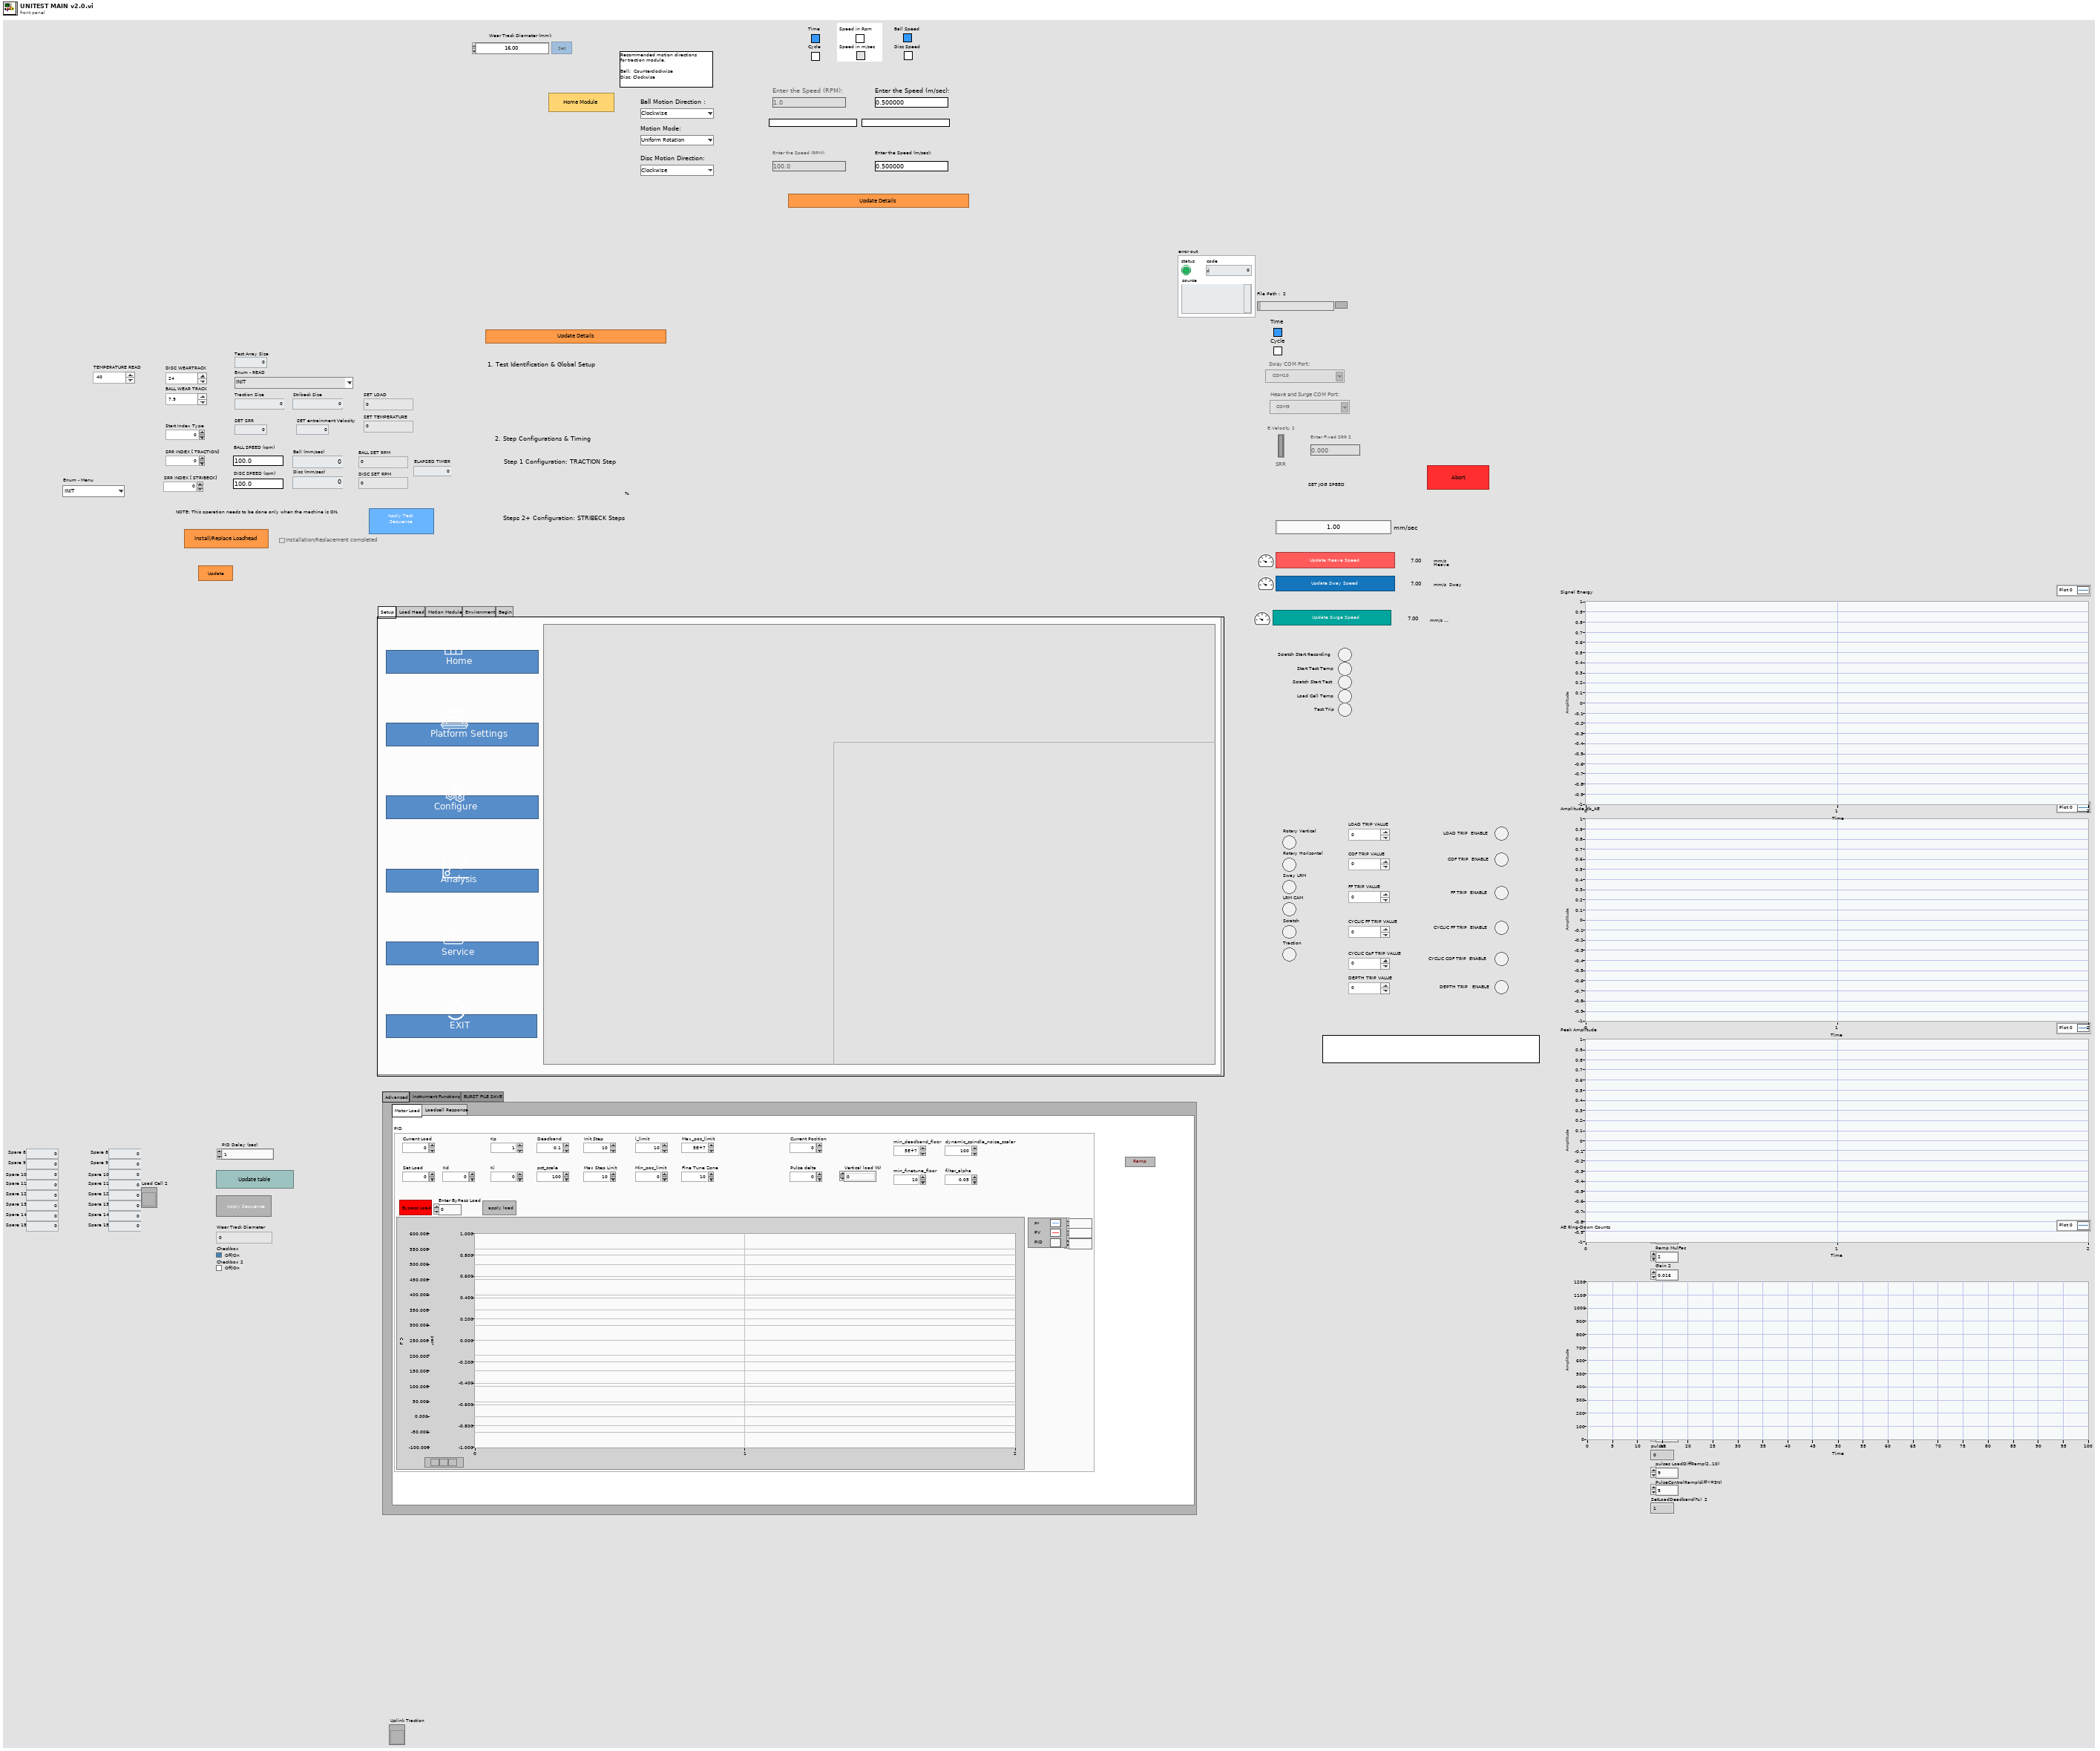
[diagram p1: front panel]
types:
  T1 = typedef "Traction Receipe Enum.ctl" = enum16{"INIT", "START", "TRACTION", "STRIBECK", "MAIN INDEX INCREMENT", "TEMPERATURE SET", "TEMPERATURE REACH", "CHURNING START", "CHURNING STOP", "LOAD", "LOAD REACHED", "SRR SET", "SRR WAIT", "SRR INCREMENT", "SPEED SET", "SPEED WAIT", "SPEED INCREMENT", "UNLOAD", "CLOSE"}
  T2 = enum32{"Uniform Rotary", "Speed Sequence", "SpeedRamp"}
  T3 = enum32{"Advanced", "Motor", "Depth_graph", "UIO Communicator", "Add to list parametrs", "Instrument Functions", "BURST FILE SAVE"}
  T4 = enum32{"LRM heating", "FBT_Heating", "Motor Load", "Loadcell Response", "Voice Load", "Step loading and speed ", "Depth"}
  T5 = cluster{"min_deadband_floor":dbl, "min_finetune_floor":dbl, "dynamic_spindle_noise_scalar":dbl, "filter_alpha":dbl, "Vertical load (N)":dbl, "Pulse delta":dbl, "Fine Tune Zone":dbl, "Max_pos_limit":dbl, "Min_pos_limit":dbl, "i_limit":dbl, "Max Step Linit":dbl, "Init Step":dbl, "pct_scale":dbl, "Deadband":dbl, "Kd":dbl, "Ki":dbl, "Kp":dbl, "Current Position":dbl, "Set Load":dbl, "Current Load":dbl, "gFF Rot 7":cluster{dbl, dbl, dbl}, "Bypass Load":bool, "Enter ByPass Load":dbl, "apply load":bool}
  T6 = cluster{"proportional gain (Kc)":dbl, "integral time (Ti, min)":dbl, "derivative time (Td, min)":dbl}
  T7 = cluster{"Sequence ID":u32, "Target Gain":u32, "Target Filter":u32, "Spare 1":u32, "Spare 2":u32, "Spare 3":u32, "Spare 4":u32, "Spare 5":u32}
  T8 = cluster{"Sequence ID":u32, "Timestamp":u32, "System Status":u32, "Peak Amplitude":sgl, "Amplitude dB_AE":sgl, "AE Ring-Down Counts":u32, "Signal Energy":sgl, "Spare 1":u32}
  T9 = cluster{"Sequence ID":u16, "Mode Command":u8, "Distance":sgl, "SPEED":sgl, "Reserved":sgl, "SPARE 1":u8, "SPARE 2":u8, "SPARE 3":u8, "SPARE 4":u8, "SPARE 5":u8, "SPARE 6":u8, "SPARE 7":u8, "SPARE 8":u8, "SPARE 9":u8, "SPARE 10":u8, "SPARE 11":u8, "SPARE 12":u8, "SPARE 13":u8, "SPARE 14":u8, "SPARE 15":u8, "SPARE 16":u8, "SPARE 17":u8}
  T10 = cluster{"Ack ID":u16, "State":u8, "Homed":u8, "HEAVE POSE":sgl, "SURGE POSE":sgl, "faultCode":u16, "fwMajor":u8, "fwMinor":u8, "Node Id":u8, "Spare 1":u8, "Spare 2":u8, "Spare 3":u8, "Spare 4":u8, "Spare 5":u8, "Spare 6":u8, "Spare 7":u8, "System UPTIME":sgl, "Missed Packets":sgl, "faultCode Heave":u16, "faultCode Surge Left":u16, "faultCode Surge Right":u16}
  T11 = cluster{"Sequence ID":u16, "Mode Command":u8, "Distance":sgl, "SPEED":sgl, "Reserved":sgl, "SPARE1":u8, "SPARE 2":u8, "SPARE  3":u8, "SPARE  4":u8, "SPARE  5":u8, "SPARE 6":u8, "SPARE 7":u8, "SPARE 8":u8, "SPARE 9":u8, "SPARE 10":u8, "SPARE 11":u8, "SPARE 12":u8, "SPARE 13":u8, "SPARE 14":u8, "SPARE 15":u8, "SPARE 16":u8, "SPARE 17":u8}
  T12 = cluster{"Ack ID ":u16, "State":u8, "Homed":u8, "SWAY POSE ":sgl, "Rotary POSE ":sgl, "faultCode":u16, "fwMajor":u8, "fwMinor":u8, "Node Id":u8, "Spare 1":u8, "Spare 2":u8, "Spare 3":u8, "Spare 4":u8, "Spare 5":u8, "Spare 6":u8, "Spare 7":u8, "System UPTIME ":sgl, "Missed Packets ":sgl, "faultCode Sway":u16, "faultCode Rotary":u16}
  T13 = cluster{"Sequence ID":u16, "Mode Command":u8, "Distance":sgl, "SPEED":sgl, "Reserved ":sgl, "SPARE 1":u8, "SPARE 2":u8, "SPARE  3":u8, "SPARE  4":u8, "SPARE  5":u8, "SPARE 6":u8, "SPARE 7":u8, "SPARE 8":u8, "SPARE 9":u8, "SPARE 10":u8, "SPARE 11":u8, "SPARE 12":u8, "SPARE 13":u8, "SPARE 14":u8, "SPARE 15":u8, "SPARE 16":u8, "SPARE 17":u8}
  T14 = cluster{"Ack ID":u16, "State":u8, "Homed":u8, "TRACTION POSE 1":sgl, "TRACTION POSE 2":sgl, "faultCode ":u16, "fwMajor ":u8, "fwMinor":u8, "Node Id":u8, "Spare 1":u8, "Spare 2":u8, "Spare 3":u8, "Spare 4":u8, "Spare 5":u8, "Spare 6":u8, "Spare 7":u8, "System UPTIME":sgl, "Missed Packets":sgl, "faultCode Traction 1":u16, "faultCode Traction 2":u16}
  T15 = enum32{"Setup", "Load Head", "Motion Module", "Environment", "Begin"}
  T16 = enum32{"Details", "PlatformSetting", "Analysis", "HOME"}
  T17 = enum32{"Constant", "Ramp", "Step", "Indentation"}
  T18 = enum32{"Uniform Rotation", "Angular Oscillation", "Speed Ramp", "Speed Step"}
  T19 = enum32{"  Acquire  ", "Compare Files Rot", "About", "Service"}
  T20 = enum32{"Coefficient of Friction ", "Friction Force (N)", "Cyclic Friction Force (N)", "Cyclic Coefficient of Friction "}
  T21 = enum32{"Speed", "Temperature", "ECR", "Acoustic Emission", "Humidity", "Sliding Distance"}
  T22 = typedef "LAB-IQ UI Data.ctl" = cluster{"Main Home Screen":cluster{"GUI":refnum<vi>, "Platform Settings":refnum<vi>, "Configure":refnum<vi>, "Home":refnum<vi>, "EXIT":refnum<vi>, "service 2":refnum<vi>, "MainPage":refnum<vi>, "Analysis":refnum<vi>}, "Platform Settings":cluster{"mm/s  Surge":refnum<vi>, "Update Surge Speed":refnum<vi>, "Drive Error":refnum<vi>, "Disable Axis Jog Soft Limits":refnum<vi>, "mm/s  Sway":refnum<vi>, "Sway and Surge COM Status":refnum<vi>, "Heave COM Status":refnum<vi>, "Enable Platform":refnum<vi>, "Surge Forward Main":refnum<vi>, "Sway Right Main":refnum<vi>, "Sway Left Main":refnum<vi>, "Heave Down Main":refnum<vi>, "Heave Up main":refnum<vi>, "Update Sway Speed":refnum<vi>, "Update Heave Speed":refnum<vi>, "mm/s Heave":refnum<vi>, "mm/sec":refnum<vi>, "mm":refnum<vi>, "Surge Backward Main":refnum<vi>}, "Analysis Screen":cluster{"Analysis Home":refnum<vi>, "Surface Analysis":refnum<vi>, "Imaging":refnum<vi>, "Image Analysis":refnum<vi>, "Post Analysis":refnum<vi>}, "Config Screen":cluster{"Select Load Head":refnum<vi>, "Notes :":refnum<vi>, "FILE":refnum<vi>, "Sample ID :":refnum<vi>, "Operator ID :":refnum<vi>, "Operator Name :":refnum<vi>, "Auto":refnum<vi>}, "Motion Module":cluster{"zNL":refnum<vi>, "NL disp":refnum<vi>, "Rotary Tab":refnum<vi>, "Motion Direction:  3":refnum<vi>, "E.Velocity 2":refnum<vi>, "e.v/ssr 2":refnum<vi>, "Enter Fixed E.Velocity 2":refnum<vi>, "Enter Final SRR 2":refnum<vi>, "Enter initial SRR 2":refnum<vi>, "Enter Fixed SRR 2":refnum<vi>, "Enter the Final E.Velocity (m/s) 2":refnum<vi>, "Enter initial E.Velocity (m/s) 2":refnum<vi>, "Final Speed (RPM) 3":refnum<vi>, "Initial Speed (RPM) 2":refnum<vi>, "Enter the Final Velocity (m/s) 3":refnum<vi>, "Enter initial Velocity (m/s)  3":refnum<vi>, "Ramp Up 2":refnum<vi>, "TEST SELECTION":refnum<vi>, "SPEED SELECTION : ":refnum<vi>, "Angular Oscillation Set":refnum<vi>, "Traction":refnum<vi>, "Step Speed":refnum<vi>, "StepTable For Load-Speed":refnum<vi>, "StepTable For Speed":refnum<vi>, "Surge Forward MM":refnum<vi>, "Surge Backward MM":refnum<vi>, "M3 Image":refnum<vi>, "String 39":refnum<vi>, "Sway Left MM":refnum<vi>, "Sway Right MM":refnum<vi>, "Disable Axis Jog Soft Limits":refnum<vi>, "mm":refnum<vi>, "Heave Down MM":refnum<vi>, "Heave Up MM":refnum<vi>, "Wear Track Diameter (mm)":refnum<vi>, "Set WTD":refnum<vi>, "HomeScratch":refnum<vi>, "HomeRot":refnum<vi>, "PlaceModule":refnum<vi>, "Enter the Angle (Deg)":refnum<vi>, "Enter the Frequency (Hz)":refnum<vi>, "Motion Mode:":refnum<vi>, "LR Sway":refnum<vi>, "Rot Hor":refnum<vi>, "Scratch":refnum<vi>, "LR Cam":refnum<vi>, "MMBack":refnum<vi>, "MMNext":refnum<vi>, "Rot Ver":refnum<vi>, "Rotary Module Selection":refnum<vi>, "calculate rotary":refnum<vi>, "SPEED SELECTION : rotary":refnum<vi>, "Import 2":refnum<vi>, "Save 2":refnum<vi>, "File Path :  2":refnum<vi>, "String 45":refnum<vi>, "StepTable For Speed 3":refnum<vi>, "Enter the Speed(mm/sec)":refnum<vi>, "Enter the Speed(RPM)":refnum<vi>, "Enter Scratch Speed (mm/s):":refnum<vi>, "SwaySpeed Set":refnum<vi>, "Scartch Offset":refnum<vi>, "Motion type:":refnum<vi>, "HomeScratch 2":refnum<vi>, "Enter Scratch length (mm):":refnum<vi>, "Wear Track Diameter":refnum<vi>, "Rotary Speed Exced":refnum<vi>, "Scratch Mode":refnum<vi>, "No of Scratch":refnum<vi>}, "Environmental control":cluster{"Humidity  Status  3":refnum<vi>, "Low Temp  Status  2":refnum<vi>, "TK4 status 2":refnum<vi>, "Stage Temperature":refnum<vi>, "Sample Temperature":refnum<vi>, "Humidity (Amb)":refnum<vi>, "Clear List":refnum<vi>, "Add to list":refnum<vi>, "Wear":refnum<vi>, "Vibration":refnum<vi>, "Humidity (Chamber)":refnum<vi>, "Temperature (Chamber)":refnum<vi>, "ECR ":refnum<vi>, "Temperature (Amb)":refnum<vi>, "Microphone":refnum<vi>, "Acoustic Emission 3":refnum<vi>, "SNext":refnum<vi>, "APBack":refnum<vi>, "Enter the Temperature (°C):":refnum<vi>, "Enter the Stage \nTemperature (°C):":refnum<vi>, "Enter the Humidity (%Rh):":refnum<vi>, "Low Temp":refnum<vi>, "High Temp":refnum<vi>, "Humidity":refnum<vi>, "Sensors Picked":refnum<vi>}, "About Screen":cluster{"Password":refnum<vi>, "Home Service":refnum<vi>, "Advanced Setting":refnum<vi>, "About Tab":refnum<vi>, "ECR Port:":refnum<vi>, "Ramp Port:":refnum<vi>, "Installation/Replacement completed":refnum<vi>, "Loahead":refnum<vi>, "Heave and Surge COM Port:":refnum<vi>, "Sway COM Port:":refnum<vi>, "Temp Modbus:":refnum<vi>, "Humidity Port:":refnum<vi>, "Edit Gain Constants":refnum<vi>, "Save Gain Constants":refnum<vi>}, "Main Screen":cluster{"Main Screen Tab":refnum<vi>, "Angle and Frequency":refnum<vi>, "Stroke (mm)":refnum<vi>, "Angle (Deg)":refnum<vi>, "Main Speed Tab":refnum<vi>, "MTM MOTOR DISPLAY":refnum<vi>, "Disc Speed (m/sec)":refnum<vi>, "Ball Speed (m/sec)":refnum<vi>, "Disc Speed (RPM)":refnum<vi>, "Ball Speed (RPM)":refnum<vi>, "SPEED TAB":refnum<vi>, "Speed (m/sec)":refnum<vi>, "Set Speed (m/sec)":refnum<vi>, "Speed (RPM)":refnum<vi>, "Set Speed":refnum<vi>, "Time Tab":refnum<vi>, "Time ( HH:MM:SS ) 2":refnum<vi>, "Test Duration":refnum<vi>, "Test Duration 4":refnum<vi>, "TEST CYCLE":refnum<vi>, "TOTAL CYCLES":refnum<vi>, "Set Load (N)":refnum<vi>, "Temp Tabs":refnum<vi>, "Heater":refnum<vi>, "TK4 status":refnum<vi>, "ChamberTemp":refnum<vi>, "SetTmp":refnum<vi>, "Controller  Status":refnum<vi>, "ChamberTemp 2":refnum<vi>, "SetTmp 2":refnum<vi>, "Controller  Status 2":refnum<vi>, "ChamberTemp 3":refnum<vi>, "SetTmp 3":refnum<vi>, "Cooling":refnum<vi>, "Load Communication":refnum<vi>, "Ambient \nTemperature":refnum<vi>, "HumCOMStatus":refnum<vi>, "Ambient\n Humidity":refnum<vi>, "Freq (Hz)":refnum<vi>, "Load En":refnum<vi>, "NLt":refnum<vi>, "zNL 2":refnum<vi>, "Humidity On":refnum<vi>, "humidity disp":refnum<vi>, "Set Humidity":refnum<vi>, "NL disp 2":refnum<vi>, "Humidity On 2":refnum<vi>, "humidity disp 2":refnum<vi>, "Set Humidity 2":refnum<vi>, "NL disp 3":refnum<vi>, "AppLoadSeq scratch":refnum<vi>, "Stop Scratch":refnum<vi>, "ClrLog":refnum<vi>, "Trip Log":refnum<vi>, "STOP":refnum<vi>, "Start Test":refnum<vi>, "Test status":refnum<vi>, "AR Led":refnum<vi>, "Data":refnum<vi>, "Health":refnum<vi>, "Sway COM Status":refnum<vi>, "Heave COM Status":refnum<vi>, "Grp Tab":refnum<vi>, "Sub Graph":refnum<vi>, "SD (mm)":refnum<vi>, "Siliding distance Reset Graph":refnum<vi>, "SDGp":refnum<vi>, "Humidity Reset Graph":refnum<vi>, "HumrGp":refnum<vi>, "Acoustic Emission (mV)":refnum<vi>, "Aqucostic Reset Graph":refnum<vi>, "gACQUOS":refnum<vi>, "ECR RESET":refnum<vi>, "ECR":refnum<vi>, "Temperature Reset":refnum<vi>, "Acoustic Emission (mV) 2":refnum<vi>, "Aqucostic Reset Graph 2":refnum<vi>, "gACQUOS 2":refnum<vi>, "ECR RESET 2":refnum<vi>, "ECR 2":refnum<vi>, "Temperature Reset 2":refnum<vi>, "Temperature (deg c)":refnum<vi>, "Speed Reset Graph":refnum<vi>, "Speed Tab":refnum<vi>, "MTM DISC  SPEED":refnum<vi>, "MTM BALL SPEED":refnum<vi>, 
